vi "UTIL_Error v1_0_0.vi"(8 "error in (no error)":errorcluster, 10 "State":string="Error", 11 "name (unnamed)":string="Error") -> (0 "error out":errorcluster)   [LabVIEW 2015]
doc: "UTIL_Error.vi\n\nThis vi Sends a command to the Error Q.vi. It will cause the Error Q.vi to put a note in the error log with a current time stamp stating the error code, error statement, and the state of the calling vi in which the error occured. \n\nNote: if the Error Q.vi is not running this will prompt the user with an error.\n\nSee Error Q.vi for futher definition of how this information is logged.\nCreated 2006 by\n\nJ. Daren Suntych\nNational Analytics\n970-397-0764"
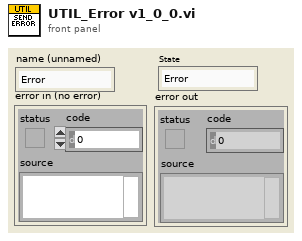
[diagram p1: front panel]
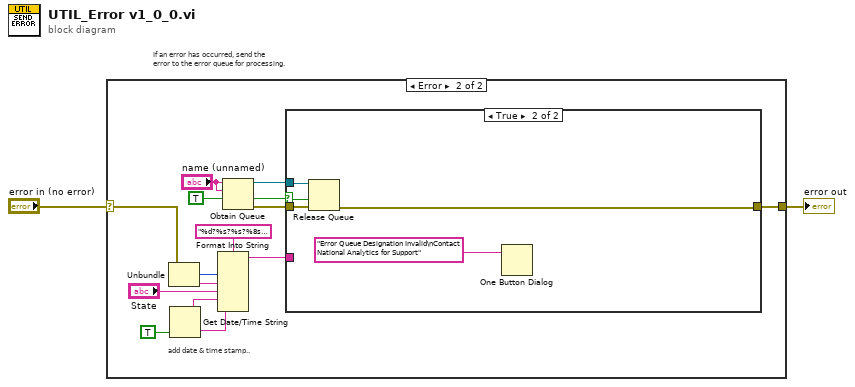
[diagram p0: block diagram]
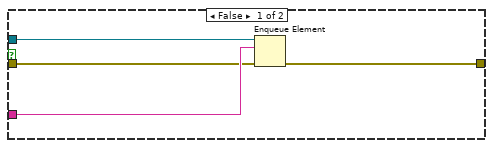
[diagram p3: hidden frame]
diagram:
  # "If an error has occurred, send the\nerror to the error queue for processing."
  n1 = case shown="Error" "error in (no error)" {
    selector: "error in (no error)" -> [w3 w12]
    tunnel: [w3 w10] -> w1
    frame No Error {
    }
    frame Error {
      # "add date & time stamp.."
      n2 = Unbundle(w12) -> ("code"=w14:i32, "source"=w13:string)  [unwired: 1 out]
      n3 = Get Date/Time String(want seconds? (F)=TRUE) -> (date string=w5:string, time string=w4:string)  [unwired: 1 in, 1 out]
      n4 = Format Into String(format string="%d?%s?%s?%8s %s", w14, w13, "State", w5, w4) -> (resulting string=w7:string)  [unwired: 2 in, 1 out]
      n5 = Obtain Queue(name (unnamed)="name (unnamed)", element data type="name (unnamed)", create if not found? (T)=TRUE) -> (queue out=w15:refnum<queue>, created new?=w9:bool, error out=w11:errorcluster)  [unwired: 2 in]
      n6 = case shown="True" w9 {
        selector: w9 -> [_ w25]
        tunnel: w7 -> [w22 _]
        tunnel: w15 -> [w21 w27]
        tunnel: w11 -> [w20 w26]
        tunnel: [w19 w24] -> w10
        frame False {
          n7 = Enqueue Element(queue=w21, element=w22, error in (no error)=w20) -> (error out=w19:errorcluster)  [unwired: 3 out]
        }
        frame True {
          n8 = Release Queue(queue=w27, force destroy? (F)=w25, error in (no error)=w26) -> (error out=w24:errorcluster)  [unwired: 2 out]
          n9 = One Button Dialog(message="Error Queue Designation Invalid\nContact National Analytics for Support" ("window title (\"\")")) -> ()  [unwired: 2 out]
        }
      }
    }
  }
  "error out" <- w1
